vi "HandleInput.vi"(7 "LoopTiming":u32, 8 "error in (no error)":errorcluster, 11 "TeleopInstruction":T1) -> (0 "error out":errorcluster)   [LabVIEW 2013]
uses:
  TeleopInstruction.ctl
panel:
  in  "Deadzone":dbl=0.1
  out "Time":u32
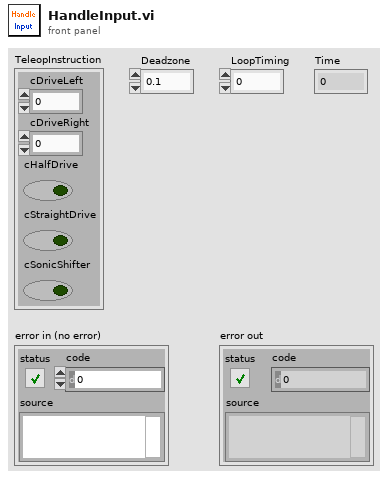
[diagram p1: front panel]
types:
  T1 = typedef "TeleopInstruction.ctl" = cluster{"cDriveLeft":dbl, "cDriveRight":dbl, "cHalfDrive":bool, "cStraightDrive":bool, "cSonicShifter":bool}
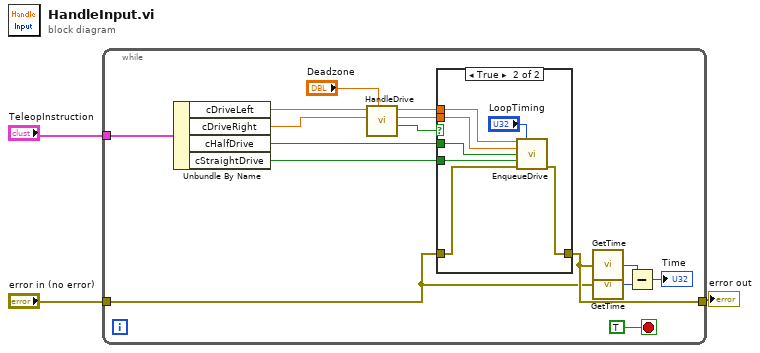
[diagram p0: block diagram]
diagram:
  n1 = while {
    tunnel: "error in (no error)" -> [w8]
    tunnel: [w17] -> w3
    tunnel: "TeleopInstruction" -> [w13]
    stop <- TRUE stop-if-true
    n2 = Unbundle By Name(w13) -> ("cDriveLeft"=w12:dbl, "cDriveRight"=w11:dbl, "cHalfDrive"=w10:bool, "cStraightDrive"=w9:bool)
    n3 = call "HandleDrive.vi"("Deadzone"="Deadzone", "RightMotor"=w11, "LeftMotor"=w12) -> ("Enqueue?"=w6:bool, "RightMotor"=w4:dbl, "LeftMotor"=w5:dbl)  [unwired: 6 in]
    n4 = case shown="True" w6 {
      tunnel: [w19 w25] -> w17
      tunnel: w8 -> [w19 w24]
      tunnel: w5 -> [_ w23]
      tunnel: w4 -> [_ w22]
      tunnel: w10 -> [_ w21]
      tunnel: w9 -> [_ w20]
      frame False {
      }
      frame True {
        n5 = call "EnqueueDrive.vi"("cDriveLeft"=w23, "LoopTiming"="LoopTiming", "cDriveRight"=w22, "cHalfDrive"=w21, "cStraightDrive"=w20, "error in (no error)"=w24) -> ("error out"=w25:errorcluster)  [unwired: 9 in]
      }
    }
    n6 = call "GetTime.vi"("error in"=w17) -> ("Time"=w16:u32)
    n7 = call "GetTime.vi"("error in"=w8) -> ("Time"=w15:u32)
    n8 = Subtract(x=w16, y=w15) -> (x-y=→"Time":u32)
  }
  "error out" <- w3
